vi "ReadWaveformSetupTrigger.vi"() -> ()   [LabVIEW 2012]
uses:
  Madlib.dll
panel:
  in  "Axis":u32
  in  "ADC Rate (ms)":dbl=1.0 min=0.033333 max=5.0 format="%.4f"
  in  "Number of Positions":u32=2 min=2 max=1000
  out "Array":dbl[](array[numeric]) format="%.4f"
  # "This example demonstrates reading a series of positions after being initiated by a trigger."
  # "X = 1\nY = 2\nZ = 3"
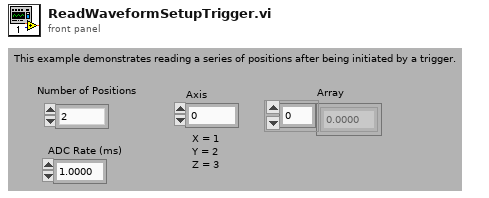
[diagram p1: front panel]
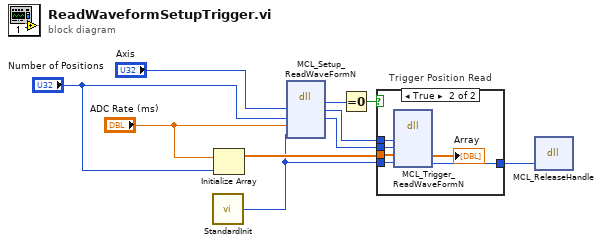
[diagram p0: block diagram]
diagram:
  n1 = call "StandardInit.vi"() -> ("Outgoing Handle"=w2:i32)  [unwired: 1 in]
  n2 = Initialize Array "Initialize Array"("ADC Rate (ms)", "Number of Positions") -> (w4:dbl[])
  n3 = dll-call lib="C:/Users/Labview/Desktop/SRR/Madlib_x64/Labview Examples/MADLib.dll" fn="MCL_Setup_ReadWaveFormN" label="Setup Position Read"("axis"="Axis", "DataPoints"="Number of Positions", "frequency"="ADC Rate (ms)", "handle"=w2) -> (w8:i32, "axis"=w6:u32, "DataPoints"=w5:u32)  [unwired: 5 in, 2 out]
  n4 = Equal To 0?(x=w8) -> (x = 0?=w7:bool)
  n5 = case "Trigger Position Read" shown="True" w7 {
    tunnel: w6 -> [_ w16]
    tunnel: w5 -> [_ w15]
    tunnel: w4 -> [_ w14]
    tunnel: w2 -> [w11 w13]
    tunnel: [w11 w12] -> w3
    frame False {
    }
    frame True {
      n6 = dll-call lib="C:/Users/Labview/Desktop/SRR/Madlib_x64/Labview Examples/MADLib.dll" fn="MCL_Trigger_ReadWaveFormN"("axis"=w16, "Datapoints"=w15, "waveform"=w14, "handle"=w13) -> ("waveform"=→"Array":dbl[], "handle"=w12:i32)  [unwired: 6 in, 2 out]
    }
  }
  n7 = dll-call lib="C:/Users/Labview/Desktop/SRR/Madlib_x64/Labview Examples/MADLib.dll" fn="MCL_ReleaseHandle"("handle"=w3) -> ()  [unwired: 5 in, 2 out]
